vi "Rio_XY_Control.vi"(8 "Error In":errorcluster, 11 "Input Cluster":T1={"X(t)/Y(f) Selection "=TRUE, "Duty Cycle (0-1) (X Control)"=0.0, "Frequency [Hz] (Y Control)"=0.0, "Direction (t:+, f:-)"=TRUE}) -> (0 "Error Out":errorcluster)   [LabVIEW 2017]
doc: "Written by Stefan Clarkson, Robin Moore & Thomas Quinn 28/02/18.\n\nThis VI takes duty cycle and freqency inputs and translates them into continuious motor movement. \nThe X motor (DC) is set at a frequency of 100 Hz and is controlled via the duty cycle input. The Y motor\nis set at a constant duty cycle of 0.5 and is controlled via the frequency input. \n\nInput Cluster Parameters: X(t)/Y(f) Selection, Duty Cycle (0-1), Frequency [Hz], Direction (t:+, f:-)."
uses:
  <vilib>/myRIO/Instrument Drivers/Onboard IO/DIO/typedefs/DIO Reference.ctl
  <vilib>/myRIO/Common/Instrument Driver Framework/Utilities/typedefs/myRIO Generic Hardware Reference.ctl
  <vilib>/myRIO/Common/Instrument Driver Framework/Utilities/typedefs/Hardware Version Enum.ctl
  <vilib>/myRIO/Common/Instrument Driver Framework/Utilities/typedefs/myRIO v1.0 Reference.ctl
  <vilib>/myRIO/Common/Instrument Driver Framework/Utilities/typedefs/Generic FPGA Reference.ctl
  <vilib>/myRIO/Common/Instrument Driver Framework/myRIO v1.0/DIO/typedefs/DIO Channels List.ctl
  <vilib>/myRIO/Common/Instrument Driver Framework/myRIO v1.0/DIO/typedefs/DIO Channels Enum.ctl
  <vilib>/userdefined/High Color/nirio_resource_hc.ctl
  <vilib>/myRIO/Instrument Drivers/Onboard IO/PWM/typedefs/PWM Reference.ctl
  <vilib>/myRIO/Common/Instrument Driver Framework/myRIO v1.0/PWM/typedefs/PWM Channels Enum.ctl
  <vilib>/myRIO/Instrument Drivers/Onboard IO/PWM/typedefs/PWM Configuration.ctl
  <vilib>/myRIO/Common/Instrument Driver Framework/Utilities/vis/Is FPGA Ref Available.vi
  <vilib>/myRIO/Common/Instrument Driver Framework/myRIO v1.0/DIO/vis/myRIO v1.1 Open DIO.vi
  <vilib>/myRIO/Instrument Drivers/Onboard IO/DIO/vis/Write.vi
  <vilib>/myRIO/Common/Instrument Driver Framework/myRIO v1.0/PWM/vis/myRIO v1.1 Open PWM.vi
  <vilib>/myRIO/Instrument Drivers/Onboard IO/PWM/vis/Set Duty Cycle and Frequency.vi
  <vilib>/myRIO/Common/Instrument Driver Framework/Utilities/vis/Validate Channels.vi
  <vilib>/myRIO/Common/Instrument Driver Framework/myRIO v1.0/DIO/vis/myRIO v1.0 Reserve DIO.vi
  <vilib>/myRIO/Common/Instrument Driver Framework/myRIO v1.0/PWM/vis/myRIO v1.0 Reserve PWM.vi
  <vilib>/myRIO/Common/Instrument Driver Framework/myRIO v1.0/Resource Manager/vis/myRIO v1.0 Reserve Channel List.vi
  <vilib>/myRIO/Common/Instrument Driver Framework/myRIO v1.0/DIO/vis/myRIO v1.0 Build MUX Configuration DIO.vi
  <vilib>/myRIO/Common/Instrument Driver Framework/myRIO v1.0/PWM/vis/myRIO v1.0 Build MUX Configuration PWM.vi
  <vilib>/myRIO/Common/Instrument Driver Framework/myRIO v1.0/Resource Manager/vis/myRIO v1.0 Reserve Channel.vi
  <vilib>/myRIO/Common/Instrument Driver Framework/myRIO v1.0/Resource Manager/vis/myRIO v1.0 Unreserve Channel.vi
  <vilib>/myRIO/Common/Instrument Driver Framework/myRIO v1.0/Resource Manager/vis/myRIO v1.0 Create Configuration List.vi
  <vilib>/myRIO/Common/Instrument Driver Framework/myRIO v1.0/Resource Manager/vis/myRIO v1.0 Build Mutex Name.vi
  <vilib>/Utility/VariantDataType/GetNumericInfo.vi
  <vilib>/Utility/error.llb/Error Cluster From Error Code.vi
  <vilib>/myRIO/Common/Instrument Driver Framework/myRIO v1.0/myRIO v1.1 Open.vi
  <vilib>/myRIO/Common/Instrument Driver Framework/Utilities/vis/IO Manager.vi
  <vilib>/myRIO/Common/Instrument Driver Framework/Utilities/vis/Configuration Manager.vi
  <vilib>/myRIO/Common/Instrument Driver Framework/myRIO v1.0/Resource Manager/vis/myRIO v1.0 Configure IO.vi
  <vilib>/myRIO/Common/Instrument Driver Framework/myRIO v1.0/myRIO v1.0 Close.vi
  <vilib>/myRIO/Common/Instrument Driver Framework/myRIO v1.0/DIO/vis/myRIO v1.0 Write DIO.vi
  <vilib>/myRIO/Common/Instrument Driver Framework/myRIO v1.0/PWM/vis/myRIO v1.0 Write PWM.vi
  <vilib>/myRIO/Express VI/Onboard IO/DO/DO Express VI.xnode
  <vilib>/myRIO/Instrument Drivers/Onboard IO/DIO/vis/myRIO DIO Open.xnode
  <vilib>/myRIO/Express VI/Onboard IO/PWM/PWM Express VI.xnode
  <vilib>/myRIO/Instrument Drivers/Onboard IO/PWM/vis/myRIO PWM Open.xnode
  <vilib>/myRIO/Instrument Drivers/Onboard IO/DIO/DIO.lvlib
  <vilib>/myRIO/Instrument Drivers/Onboard IO/PWM/PWM.lvlib
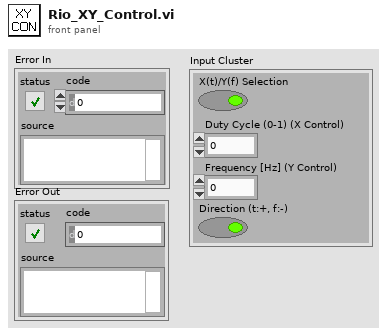
[diagram p1: front panel]
types:
  T1 = cluster{"X(t)/Y(f) Selection ":bool, "Duty Cycle (0-1) (X Control)":dbl, "Frequency [Hz] (Y Control)":dbl, "Direction (t:+, f:-)":bool}
  T2 = typedef "DIO.lvlib/DIO Reference.ctl" = cluster{"myRIO Reference":T3, "DIO Channels List":T7}
  T3 = typedef "myRIO Generic Hardware Reference.ctl" = cluster{"myRIO Model":T4, "myRIO Hardware Reference":T5}
  T4 = typedef "Hardware Version Enum.ctl" = enum16{"Unknown", "myRIO-1900", "myRIO-1950", "roboRIO", "NI ELVIS RIO CM"}
  T5 = typedef "myRIO v1.0 Reference.ctl" = cluster{"Generic FPGA Reference":T6, "Allow multiple opens":bool}
  T6 = typedef "Generic FPGA Reference.ctl" = refnum<k20>
  T7 = typedef "DIO Channels List.ctl" = T8[]
  T8 = typedef "DIO Channels Enum.ctl" = enum16{"Not Connected", "C/DIO0", "C/DIO1", "C/DIO2", "C/DIO3", "C/DIO4", "C/DIO5", "C/DIO6", "C/DIO7", "A/DIO0", "A/DIO1", "A/DIO2", "A/DIO3", "A/DIO4", "A/DIO5", "A/DIO6", "A/DIO7", "A/DIO8", "A/DIO9", "A/DIO10", "A/DIO11", "A/DIO12", "A/DIO13", "A/DIO14", "A/DIO15", "B/DIO0", "B/DIO1", "B/DIO2", "B/DIO3", "B/DIO4", "B/DIO5", "B/DIO6", "B/DIO7", "B/DIO8", "B/DIO9", "B/DIO10", "B/DIO11", "B/DIO12", "B/DIO13", "B/DIO14", "B/DIO15", "LED0", "LED1", "LED2", "LED3", "Button0", "DIO/DIO0", "DIO/DIO1", "DIO/DIO2", "DIO/DIO3", "DIO/DIO4", "DIO/DIO5", "DIO/DIO6", "DIO/DIO7", "DIO/DIO8", "DIO/DIO9", "SPI/CS0", "SPI/CS1", "SPI/CS2", "SPI/CS3", "LED RADIO (Green)", "LED RADIO (Red)", "LED COMM (Green)", "LED COMM (Red)", "LED MODE (Green)", "LED MODE (Red)"}
  T9 = typedef "nirio_resource_hc.ctl" = tag
  T10 = typedef "PWM.lvlib/PWM Reference.ctl" = cluster{"myRIO Reference":T3, "PWM Channels Enum":T11, "PWM Configuration":T12}
  T11 = typedef "PWM Channels Enum.ctl" = enum16{"Not Connected", "C/PWM0", "C/PWM1", "A/PWM0", "A/PWM1", "A/PWM2", "B/PWM0", "B/PWM1", "B/PWM2", "PWM/PWM0", "PWM/PWM1", "PWM/PWM2", "PWM/PWM3", "PWM/PWM4", "PWM/PWM5", "PWM/PWM6", "PWM/PWM7", "PWM/PWM8", "PWM/PWM9"}
  T12 = typedef "PWM.lvlib/PWM Configuration.ctl" = cluster{"Frequency":dbl, "Duty Cycle":dbl}
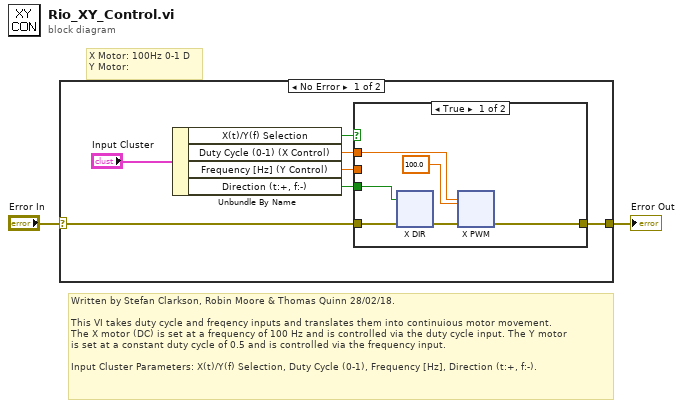
[diagram p0: block diagram]
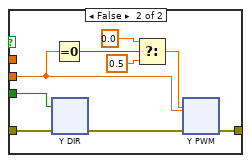
[diagram p2: hidden frame]
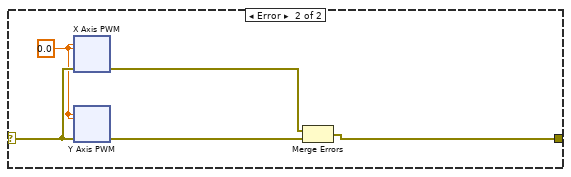
[diagram p3: hidden frame]
diagram:
  # "Written by Stefan Clarkson, Robin Moore & Thomas Quinn 28/02/18.\n\nThis VI takes duty cycle and freqency inputs and translates them into continuious motor movement. \nThe X motor (DC) is set at a frequency of 100 Hz and is controlled via the duty cycle input. The Y motor\nis set at a constant duty cycle of 0.5 and is controlled via the frequency input. \n\nInput Cluster Parameters: X(t)/Y(f) Selection, Duty Cycle (0-1), Frequency [Hz], Direction (t:+, f:-)."
  # "X Motor: 100Hz 0-1 D\nY Motor:"
  n1 = case shown="No Error" "Error In" {
    selector: "Error In" -> [w9 w169]
    tunnel: [w8 w167] -> w1
    frame No Error {
      n2 = Unbundle By Name("Input Cluster") -> ("X(t)/Y(f) Selection"=w6:bool, "Duty Cycle (0-1) (X Control)"=w5:dbl, "Frequency [Hz] (Y Control)"=w4:dbl, "Direction (t:+, f:-)"=w3:bool)
      n3 = case shown="True" w6 {
        tunnel: w5 -> [w10 _]
        tunnel: w3 -> [w15 w87]
        tunnel: w4 -> [_ w89]
        tunnel: w9 -> [w14 w88]
        tunnel: [w12 w86] -> w8
        frame True {
          n4 = xnode "X DIR"("error in (no error)"=w14, "X Axis Direction (A/DIO4 (Pin 19))"=w15) -> ("error out"=w13:errorcluster)
          n5 = xnode "X PWM"("error in (no error)"=w13, "Duty Cycle"=w10, "Frequency [Hz]"=100.0) -> ("error out"=w12:errorcluster)
        }
        frame False {
          n6 = xnode "Y DIR"("error in (no error)"=w88, "Y Axis Direction (A/DIO5 (Pin 21))"=w87) -> ("error out"=w94:errorcluster)
          n7 = Equal To 0?(x=w89) -> (x = 0?=w92:bool)
          n8 = Select(t=0.0, s=w92, f=0.5) -> (s? t:f=w93:dbl)
          n9 = xnode "Y PWM"("error in (no error)"=w94, "Duty Cycle"=w93, "Frequency [Hz]"=w89) -> ("error out"=w86:errorcluster)
        }
      }
    }
    frame Error {
      w168 = 0.0 ("Duty Cycle")
      n10 = xnode "X Axis PWM"("error in (no error)"=w169, "Duty Cycle"=w168, "Frequency [Hz]"=w168) -> ("error out"=w166:errorcluster)
      n11 = xnode "Y Axis PWM"("error in (no error)"=w169, "Duty Cycle"=w168, "Frequency [Hz]"=w168) -> ("error out"=w165:errorcluster)
      n12 = Merge Errors(w166, w165) -> (w167:errorcluster)
    }
  }
  "Error Out" <- w1
